vi "Initialize.vi"(8 "error in (no error)":errorcluster, 9 "id query (False)":bool caption="id query (True)", 10 "reset device (False)":bool caption="reset device (True)", 11 "NiDaqMx in":refnum<class "NiDaqMx.lvclass">) -> (0 "error out":errorcluster, 3 "NiDaqMx out":refnum<class "NiDaqMx.lvclass">)   [LabVIEW 2018, in "DigitizerPlugins.lvlib" / "NiDaqMx.lvclass"]
uses:
  NiDaqMx.lvclass
  X:/Projects/PMUCal/Modules/Digitizer/DigitizerPlugins/DigitizerBaseClass/DigitizerBase.lvclass
  DigitizerBaseClass/DigitizerBase.lvclass/DigitizerBase.ctl
  DigitizerBaseClass/Accessors/Read Handle.vi
  DigitizerBaseClass/Accessors/Read InstRef.vi
  DigitizerBaseClass/Accessors/Read Channels.vi
  DigitizerBaseClass/Accessors/Write InstRef.vi
  DigitizerBaseClass/Accessors/Write Waveforms.vi
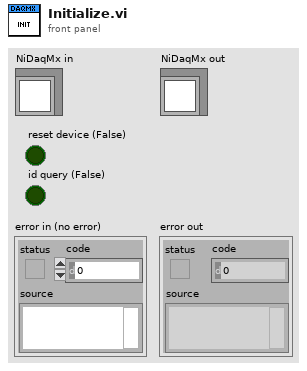
[diagram p1: front panel]
types:
  T1 = typedef "DigitizerPlugins.lvlib/DigitizerBase.lvclass/Channel.ctl" = cluster{"Name":string, "Enabled":bool, "InputImpedance":dbl, "Coupling":enum16{"AC", "DC", "Gnd"}, "Offset":dbl, "Range":dbl}
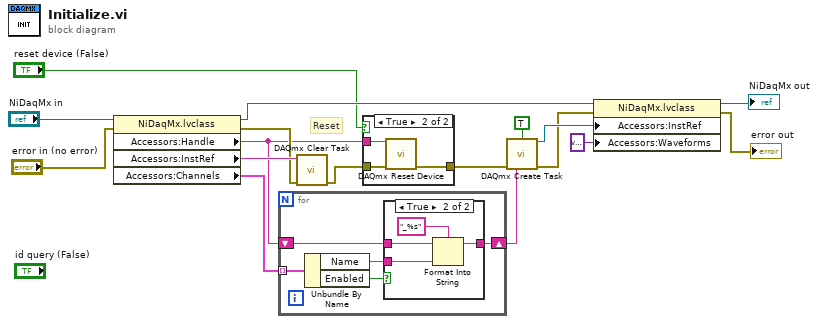
[diagram p0: block diagram]
diagram:
  # "Reset"
  n1 = property class="NiDaqMx.lvclass"(reference="NiDaqMx in", error in="error in (no error)") -> (reference out=w7:refnum<class "NiDaqMx.lvclass">, error out=w14:errorcluster, "Accessors:Handle"=w11:string, "Accessors:InstRef"=w16:string, "Accessors:Channels"=w12:T1[])
  n2 = for {
    tunnel: w12 -> [w22] mode=indexing
    shift-right: [w21] -> w10
    shift-left: w11 -> [w20]
    n3 = Unbundle By Name(w22) -> ("Name"=w19:string, "Enabled"=w18:bool)
    n4 = case shown="True" w18 {
      tunnel: [w23 w27] -> w21
      tunnel: w20 -> [w23 w26]
      tunnel: w19 -> [_ w24]
      frame False {
      }
      frame True {
        n5 = Format Into String(format string="_%s", initial string=w26, w24) -> (resulting string=w27:string)  [unwired: 1 in, 1 out]
      }
    }
  }
  n6 = call <vilib>:"DAQmx Clear Task.vi"("task in"=w16, "error in"=w14) -> ("error out"=w13:errorcluster)  [unwired: 13 in]
  n7 = case shown="True" "reset device (False)" {
    tunnel: w13 -> [w28 w31]
    tunnel: w11 -> [_ w30]
    tunnel: [w28 w29] -> w8
    frame False {
    }
    frame True {
      n8 = call <vilib>:"DAQmx Reset Device.vi"("device in"=w30, "error in"=w31) -> ("error out"=w29:errorcluster)  [unwired: 13 in]
    }
  }
  n9 = call <vilib>:"DAQmx Create Task.vi"("new task name"=w10, "auto cleanup"=TRUE, "error in"=w8) -> ("task out"=w6:refnum<k21>, "error out"=w4:errorcluster)  [unwired: 11 in]
  n10 = property class="NiDaqMx.lvclass"(reference=w7, error in=w4, "Accessors:InstRef"=w6, "Accessors:Waveforms"=variant ("Waveforms")) -> (reference out=→"NiDaqMx out":refnum<class "NiDaqMx.lvclass">, error out=→"error out":errorcluster)
